vi "Assert Single Element.vi"(8 "error in (no error)":errorcluster, 10 "Elements":refnum<class "Config Element.lvclass">[](array[class])) -> (0 "error out":errorcluster, 2 "Element":refnum<class "Config Element.lvclass">)   [LabVIEW 2020, in "CDM-Config.lvlib" / "Config Manager.lvclass"]
uses:
  Config Manager.lvclass
  Config Element/Config Element.lvclass
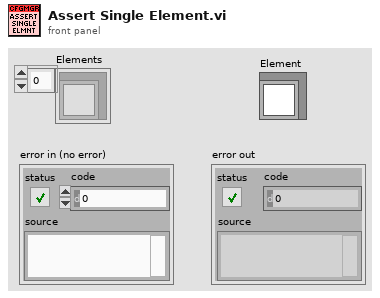
[diagram p1: front panel]
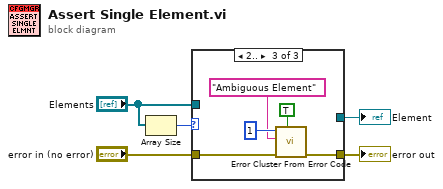
[diagram p0: block diagram]
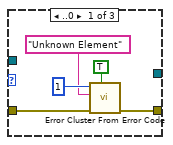
[diagram p2: hidden frame]
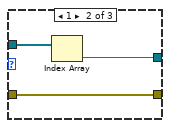
[diagram p3: hidden frame]
diagram:
  n1 = Array Size(array="Elements") -> (size(s)=w5:i32)
  n2 = case shown="2.." w5 {
    tunnel: "Elements" -> [_ w13 _]
    tunnel: [_ w12 _] -> w3
    tunnel: [w10 w11 w17] -> w2
    tunnel: "error in (no error)" -> [w8 w11 w18]
    frame ..0 {
      n3 = call <vilib>:"Error Cluster From Error Code.vi"("show call chain? (False)"=TRUE, "error in (no error)"=w8, "error message (\"\")"="Unknown Element", "error code (0)"=1) -> ("error out"=w10:errorcluster)  [unwired: 5 in]
    }
    frame 1 {
      n4 = Index Array(array=w13) -> (element=w12:refnum<class "Config Element.lvclass">)  [unwired: 1 in]
    }
    frame 2.. {
      n5 = call <vilib>:"Error Cluster From Error Code.vi"("show call chain? (False)"=TRUE, "error in (no error)"=w18, "error message (\"\")"="Ambiguous Element", "error code (0)"=1) -> ("error out"=w17:errorcluster)  [unwired: 5 in]
    }
  }
  "Element" <- w3
  "error out" <- w2
